vi "RT_Angle_Of_Attack_in_DLR_Navigation_Reference_System_vcomp(SubVI).vi"(4 "Euler Angles [rad]":cluster{"phi":dbl, "theta":dbl, "psi":dbl}, 6 "q":dbl[](array[numeric]), 8 "i":i32, 9 "V_wind [m/s]":dbl[][](array[numeric]), 10 "V (m/s)":dbl[](array[numeric]), 11 "Civita?":bool) -> (0 "Speed_direction [rad]":dbl[](array[numeric]), 2 "AoA_yaw (rad)":dbl, 3 "AoA_pitch (rad)":dbl)   [LabVIEW 2017]
uses:
  <vilib>/Analysis/coordinate.llb/Euler Rotation Order.ctl
  <vilib>/Analysis/_algsub.llb/Vector Norm Type.ctl
  <vilib>/Analysis/_algsub.llb/Real Vector Norm.vi
  <vilib>/Analysis/NI_AALPro.lvlib
panel:
  out "Elevation [deg]":dbl
  out "Azimuth [deg]":dbl
  out "appended array":dbl[](array[numeric])
  out "Speed_quat":dbl[](array[numeric])
  out "Speed_pitch (rad)":dbl
  out "Speed_yaw (rad)":dbl
  out "v":dbl[](array[numeric])
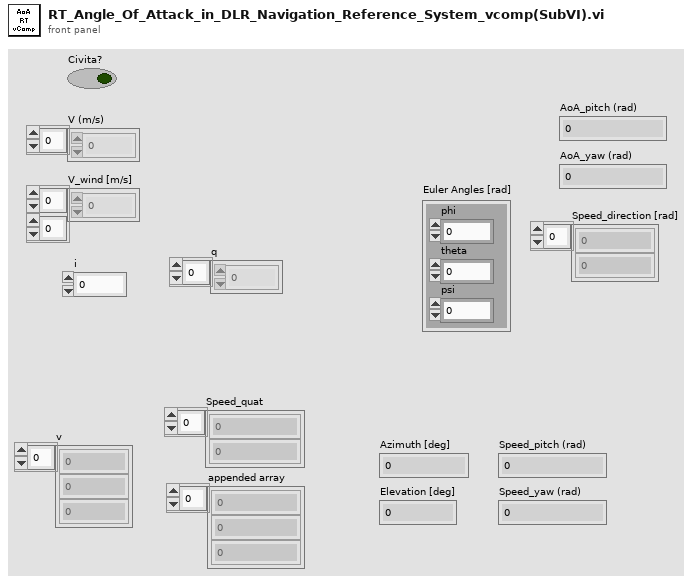
[diagram p1: front panel]
types:
  T1 = typedef "NI_AALPro.lvlib/Euler Rotation Order.ctl" = u16
  T2 = typedef "NI_AALPro.lvlib/Vector Norm Type.ctl" = u16
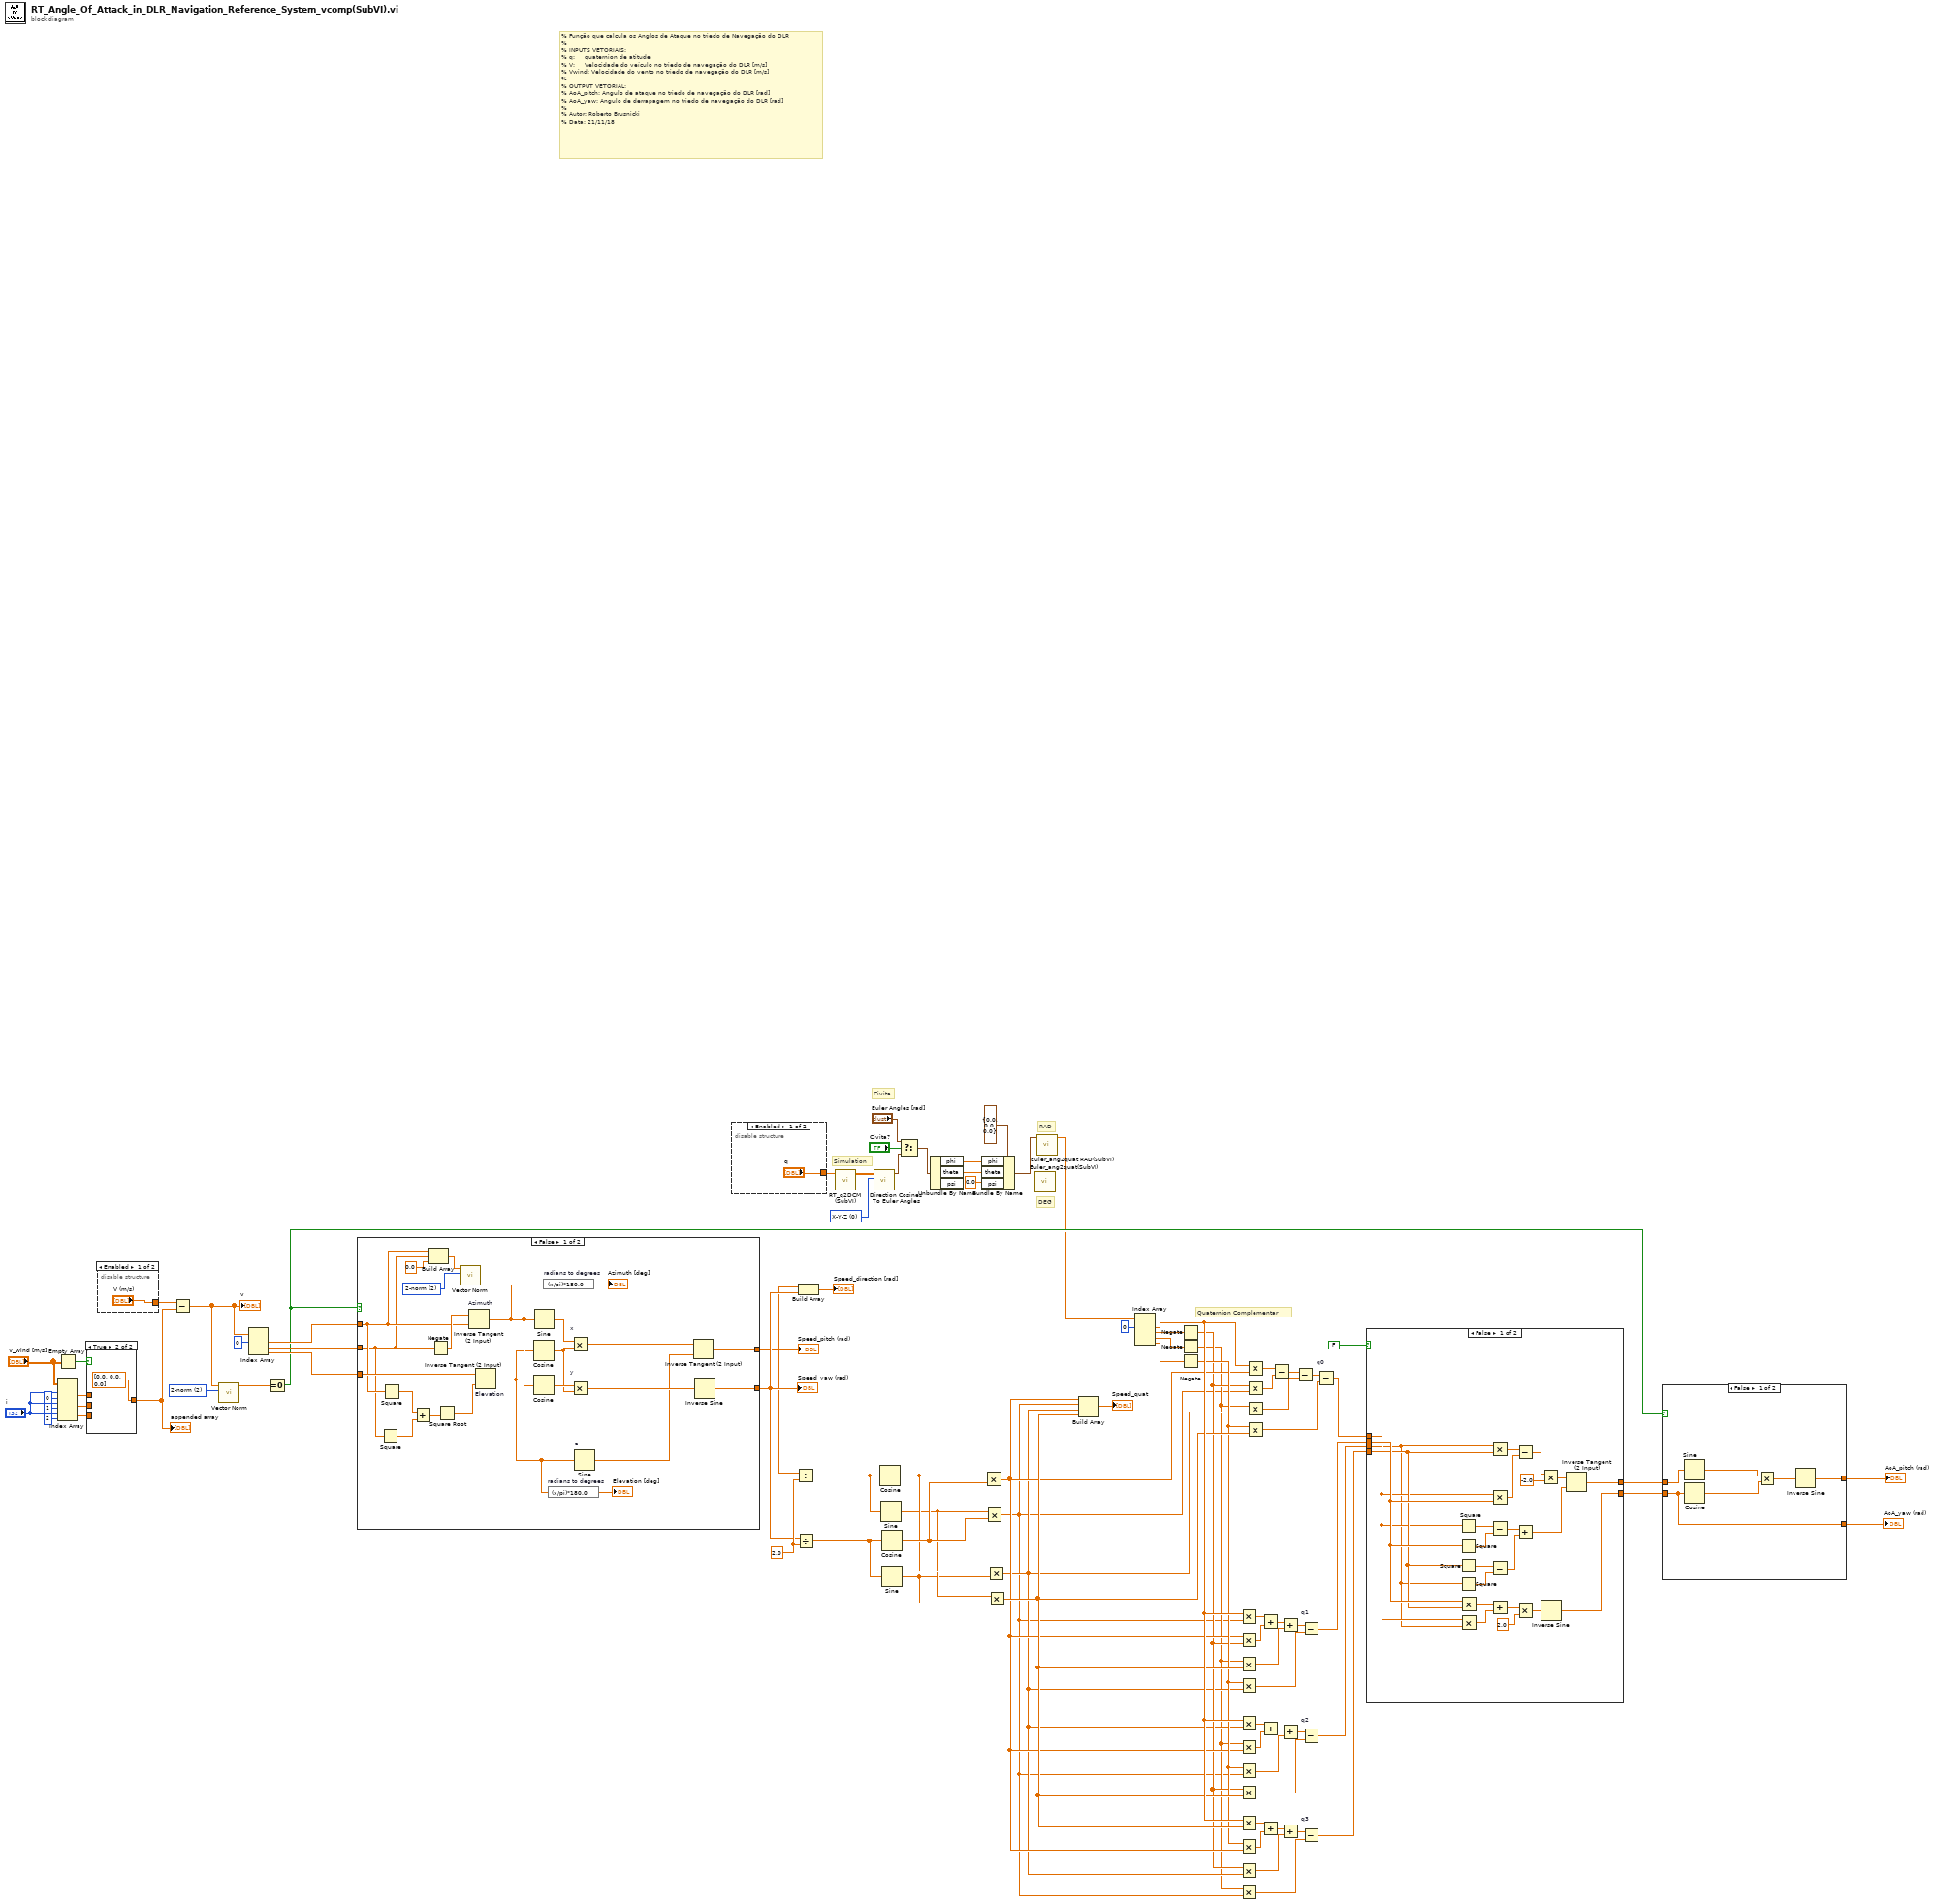
[diagram p0: block diagram]
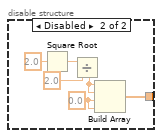
[diagram p2: hidden frame]
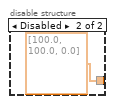
[diagram p3: hidden frame]
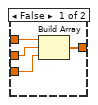
[diagram p4: hidden frame]
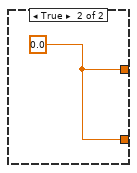
[diagram p5: hidden frame]
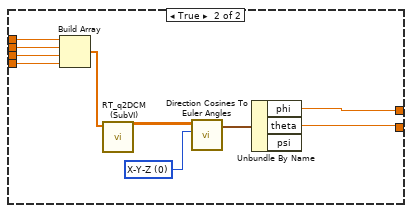
[diagram p6: hidden frame]
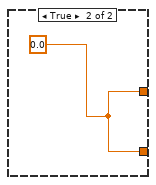
[diagram p7: hidden frame]
diagram:
  w16 = T1 0 items=["X-Y-Z", "X-Z-Y", "Y-X-Z", "Y-Z-X", "Z-X-Y", "Z-Y-X", "X-Y-X", "X-Z-X", "Y-X-Y", "Y-Z-Y", "Z-X-Z", "Z-Y-Z"] ("rotation order")
  w73 = 2.0 ("y")
  w79 = T2 2 items=["1-norm"=1, "2-norm"=2, "Inf-norm"=3, "-Inf-norm"=4, "User Defined"=5] ("norm type")
  # "DEG"
  # "RAD"
  # "Quaternion Complementar"
  # "Simulation"
  # "Civita"
  # "% Função que calcula os Anglos de Ataque no triedo de Navegação do DLR \n%\n% INPUTS VETORIAIS: \n% q:     quaternion de atitude   \n% V:     Velocidade do veículo no triedo de navegação do DLR [m/s]\n% Vwind: Velocidade do vento no triedo de navegação do DLR [m/s]\n%\n% OUTPUT VETORIAL:\n% AoA_pitch: Angulo de ataque no triedo de navegação do DLR [rad]\n% AoA_yaw: Angulo de derrapagem no triedo de navegação do DLR [rad]\n%\n% Autor: Roberto Brusnicki\n% Data: 21/11/18"
  n1 = Index Array(array="V_wind [m/s]", index (row) #1="i", index (col) #1=0 ("disabled index (col)"), index (row) #2="i", index (col) #2=1 ("disabled index (col)"), index (row) #3="i", index (col) #3=2 ("disabled index (col)")) -> (element #1=w82:dbl, element #2=w81:dbl, element #3=w80:dbl)
  n2 = Empty Array?(array="V_wind [m/s]") -> (empty?=w12:bool)
  n3 = case shown="True" w12 {
    tunnel: w82 -> [w92 _]
    tunnel: w81 -> [w91 _]
    tunnel: w80 -> [w90 _]
    tunnel: [w89 dbl[] [0.0, 0.0, 0.0]] -> w8
    frame False {
      n4 = Build Array(w92, w91, w90) -> (w89:dbl[])
    }
    frame True {
    }
  }
  "appended array" <- w8
  n5 = disable-structure shown="Enabled" {
    disable-tunnel: ["V (m/s)" dbl[] [100.0, 100.0, 0.0] ("V (m/s)")] -> w87
    frame Enabled {
    }
    frame Disabled {
    }
  }
  n6 = Subtract(x=w87, y=w8) -> (x-y=w78:dbl[])
  "v" <- w78
  n7 = call-poly <vilib>:"Vector Norm.vi"("norm type"=w79, "Input Vector"=w78) -> ("norm"=w75:dbl)  [unwired: 8 in, 1 out]
  n8 = Index Array(array=w78, index #1=0 ("index (row)")) -> (element #1=w77:dbl, element #2=w76:dbl, element #3=w22:dbl)  [unwired: 2 in]
  n9 = Equal To 0?(x=w75) -> (x = 0?=w20:bool)
  n10 = case shown="False" w20 {
    tunnel: [w109 w119] -> w72
    tunnel: [w106 w119] -> w71
    tunnel: w77 -> [w99 _]
    tunnel: w76 -> [w98 _]
    tunnel: w22 -> [w117 _]
    frame False {
      w116 = T2 2 items=["1-norm"=1, "2-norm"=2, "Inf-norm"=3, "-Inf-norm"=4, "User Defined"=5] ("norm type")
      n11 = Square(x=w98) -> (x^2=w101:dbl)
      n12 = Square(x=w99) -> (x^2=w100:dbl)
      n13 = Add(x=w100, y=w101) -> (x+y=w97:dbl)
      n14 = Build Array(w99, w98, 0.0 ("element")) -> (w114:dbl[])
      n15 = Negate(x=w98) -> (-x=w118:dbl)
      n16 = Square Root(x=w97) -> (sqrt(x)=w96:dbl)
      n17 = call-poly <vilib>:"Vector Norm.vi"("norm type"=w116, "Input Vector"=w114) -> ()  [unwired: 8 in, 2 out]
      n18 = Inverse Tangent (2 Input) "Azimuth"(1:w99, 2:w118) -> (0:w105:dbl)
      n19 = Inverse Tangent (2 Input) "Elevation"(1:w96, 2:w117) -> (0:w102:dbl)
      n20 = Cosine(x=w102) -> (cos(x)=w111:dbl)
      n21 = Cosine(x=w105) -> (cos(x)=w112:dbl)
      n22 = Sine(x=w105) -> (sin(x)=w113:dbl)
      n23 = expression code="(x/pi)*180.0" "radians to degrees"(w105) -> (→"Azimuth [deg]":dbl)
      n24 = expression code="(x/pi)*180.0" "radians to degrees"(w102) -> (→"Elevation [deg]":dbl)
      n25 = Multiply "x"(x=w113, y=w111) -> (x*y=w108:dbl)
      n26 = Multiply "y"(x=w112, y=w111) -> (x*y=w110:dbl)
      n27 = Sine "z"(x=w102) -> (sin(x)=w107:dbl)
      n28 = Inverse Tangent (2 Input)(1:w107, 2:w108) -> (0:w106:dbl)
      n29 = Inverse Sine(1:w110) -> (0:w109:dbl)
    }
    frame True {
      w119 = 0.0 ("Speed_pitch (rad)")
    }
  }
  "Speed_pitch (rad)" <- w71
  "Speed_yaw (rad)" <- w72
  n30 = disable-structure shown="Enabled" {
    disable-tunnel: ["q" w126] -> w14
    frame Enabled {
    }
    frame Disabled {
      w121 = 0.0 ("element")
      n31 = Square Root(x=2.0) -> (sqrt(x)=w124:dbl)
      n32 = Divide(x=w124, y=2.0) -> (x/y=w122:dbl)
      n33 = Build Array(w122, w122, w121, w121) -> (w126:dbl[])
    }
  }
  n34 = Divide(x=w71, y=w73) -> (x/y=w70:dbl)
  n35 = Divide(x=w72, y=w73) -> (x/y=w69:dbl)
  n36 = Build Array(w71, w72) -> (→"Speed_direction [rad]":dbl[])
  n37 = call "RT_q2DCM (SubVI).vi"("Quaternion"=w14) -> ("DCM"=w15:dbl[][])  [unwired: 10 in]
  n38 = call <vilib>:"Direction Cosines To Euler Angles.vi"("rotation order"=w16, "Direction Cosines"=w15) -> ("Euler Angles"=w4:cluster{"phi":dbl, "theta":dbl, "psi":dbl})  [unwired: 8 in, 1 out]
  n39 = Cosine(x=w70) -> (cos(x)=w67:dbl)
  n40 = Sine(x=w70) -> (sin(x)=w66:dbl)
  n41 = Cosine(x=w69) -> (cos(x)=w68:dbl)
  n42 = Sine(x=w69) -> (sin(x)=w65:dbl)
  n43 = Select(t="Euler Angles [rad]", s="Civita?", f=w4) -> (s? t:f=w2:cluster{"phi":dbl, "theta":dbl, "psi":dbl})
  n44 = Unbundle By Name(w2) -> ("phi"=w10:dbl, "theta"=w11:dbl)  [unwired: 1 out]
  n45 = Bundle By Name(cluster=cluster{"phi":dbl, "theta":dbl, "psi":dbl} {"phi"=0.0, "theta"=0.0, "psi"=0.0} ("Euler Angles 2"), "phi"=w10, "theta"=w11, "psi"=0.0) -> (w6:cluster{"phi":dbl, "theta":dbl, "psi":dbl})
  n46 = Multiply(x=w67, y=w68) -> (x*y=w33:dbl)
  n47 = Multiply(x=w66, y=w68) -> (x*y=w29:dbl)
  n48 = Multiply(x=w67, y=w65) -> (x*y=w31:dbl)
  n49 = Multiply(x=w66, y=w65) -> (x*y=w35:dbl)
  n50 = call "Euler_ang2quat(SubVI).vi"() -> ()  [unwired: 11 in, 1 out]
  n51 = call "Euler_ang2quat RAD(SubVI).vi"("Euler Angles [rad]"=w6) -> ("Quaternions"=w5:dbl[])  [unwired: 10 in]
  n52 = Build Array(w33, w29, w31, w35) -> (→"Speed_quat":dbl[])
  n53 = Index Array(array=w5, index #1=0 ("index")) -> (element #1=w36:dbl, element #2=w61:dbl, element #3=w62:dbl, element #4=w63:dbl)  [unwired: 3 in]
  n54 = Negate(x=w61) -> (-x=w32:dbl)
  n55 = Negate(x=w62) -> (-x=w30:dbl)
  n56 = Negate(x=w63) -> (-x=w34:dbl)
  n57 = Multiply(x=w36, y=w29) -> (x*y=w54:dbl)
  n58 = Multiply(x=w33, y=w32) -> (x*y=w53:dbl)
  n59 = Multiply(x=w30, y=w35) -> (x*y=w50:dbl)
  n60 = Multiply(x=w34, y=w31) -> (x*y=w49:dbl)
  n61 = Multiply(x=w36, y=w31) -> (x*y=w43:dbl)
  n62 = Multiply(x=w30, y=w33) -> (x*y=w44:dbl)
  n63 = Multiply(x=w34, y=w29) -> (x*y=w47:dbl)
  n64 = Multiply(x=w32, y=w35) -> (x*y=w48:dbl)
  n65 = Multiply(x=w36, y=w35) -> (x*y=w42:dbl)
  n66 = Multiply(x=w34, y=w33) -> (x*y=w41:dbl)
  n67 = Multiply(x=w32, y=w31) -> (x*y=w38:dbl)
  n68 = Multiply(x=w30, y=w29) -> (x*y=w37:dbl)
  n69 = Multiply(x=w36, y=w33) -> (x*y=w60:dbl)
  n70 = Multiply(x=w32, y=w29) -> (x*y=w59:dbl)
  n71 = Multiply(x=w30, y=w31) -> (x*y=w57:dbl)
  n72 = Multiply(x=w34, y=w35) -> (x*y=w55:dbl)
  n73 = Add(x=w54, y=w53) -> (x+y=w52:dbl)
  n74 = Add(x=w43, y=w44) -> (x+y=w45:dbl)
  n75 = Add(x=w42, y=w41) -> (x+y=w40:dbl)
  n76 = Subtract(x=w60, y=w59) -> (x-y=w58:dbl)
  n77 = Add(x=w52, y=w50) -> (x+y=w51:dbl)
  n78 = Add(x=w45, y=w47) -> (x+y=w46:dbl)
  n79 = Add(x=w40, y=w38) -> (x+y=w39:dbl)
  n80 = Subtract(x=w58, y=w57) -> (x-y=w56:dbl)
  n81 = Subtract "q1"(x=w51, y=w49) -> (x-y=w27:dbl)
  n82 = Subtract "q2"(x=w46, y=w48) -> (x-y=w26:dbl)
  n83 = Subtract "q3"(x=w39, y=w37) -> (x-y=w25:dbl)
  n84 = Subtract "q0"(x=w56, y=w55) -> (x-y=w28:dbl)
  n85 = case shown="False" FALSE {
    tunnel: w28 -> [w134 w159]
    tunnel: w27 -> [w136 w158]
    tunnel: w26 -> [w133 w157]
    tunnel: w25 -> [w135 w156]
    tunnel: [w137 w154] -> w24
    tunnel: [w127 w153] -> w23
    frame False {
      n86 = Square(x=w134) -> (x^2=w144:dbl)
      n87 = Square(x=w136) -> (x^2=w143:dbl)
      n88 = Square(x=w135) -> (x^2=w142:dbl)
      n89 = Square(x=w133) -> (x^2=w141:dbl)
      n90 = Multiply(x=w136, y=w135) -> (x*y=w132:dbl)
      n91 = Multiply(x=w134, y=w133) -> (x*y=w131:dbl)
      n92 = Multiply(x=w133, y=w135) -> (x*y=w149:dbl)
      n93 = Multiply(x=w134, y=w136) -> (x*y=w148:dbl)
      n94 = Subtract(x=w144, y=w143) -> (x-y=w140:dbl)
      n95 = Subtract(x=w142, y=w141) -> (x-y=w139:dbl)
      n96 = Add(x=w132, y=w131) -> (x+y=w129:dbl)
      n97 = Subtract(x=w149, y=w148) -> (x-y=w147:dbl)
      n98 = Add(x=w140, y=w139) -> (x+y=w138:dbl)
      n99 = Multiply(x=w129, y=2.0) -> (x*y=w128:dbl)
      n100 = Multiply(x=w147, y=-2.0) -> (x*y=w145:dbl)
      n101 = Inverse Sine(1:w128) -> (0:w127:dbl)
      n102 = Inverse Tangent (2 Input)(1:w138, 2:w145) -> (0:w137:dbl)
    }
    frame True {
      w151 = T1 0 items=["X-Y-Z", "X-Z-Y", "Y-X-Z", "Y-Z-X", "Z-X-Y", "Z-Y-X", "X-Y-X", "X-Z-X", "Y-X-Y", "Y-Z-Y", "Z-X-Z", "Z-Y-Z"] ("rotation order")
      n103 = Build Array(w159, w158, w157, w156) -> (w155:dbl[])
      n104 = call "RT_q2DCM (SubVI).vi"("Quaternion"=w155) -> ("DCM"=w152:dbl[][])  [unwired: 10 in]
      n105 = call <vilib>:"Direction Cosines To Euler Angles.vi"("rotation order"=w151, "Direction Cosines"=w152) -> ("Euler Angles"=w150:cluster{"phi":dbl, "theta":dbl, "psi":dbl})  [unwired: 8 in, 1 out]
      n106 = Unbundle By Name(w150) -> ("phi"=w154:dbl, "theta"=w153:dbl)  [unwired: 1 out]
    }
  }
  n107 = case shown="False" w20 {
    tunnel: w24 -> [w165 _]
    tunnel: [w161 w166] -> w19
    tunnel: w23 -> [w160 _]
    tunnel: [w160 w166] -> w18
    frame False {
      n108 = Sine(x=w165) -> (sin(x)=w164:dbl)
      n109 = Cosine(x=w160) -> (cos(x)=w163:dbl)
      n110 = Multiply(x=w164, y=w163) -> (x*y=w162:dbl)
      n111 = Inverse Sine(1:w162) -> (0:w161:dbl)
    }
    frame True {
      w166 = 0.0
    }
  }
  "AoA_pitch (rad)" <- w19
  "AoA_yaw (rad)" <- w18
